vi "goInCircles.vi"(8 "error in (no error)":errorcluster, 11 "StationKeeping in":refnum<class "StationKeeping.lvclass">) -> (0 "error out":errorcluster, 2 "No Sail Circles":T1[](array[typedef]), 3 "StationKeeping out":refnum<class "StationKeeping.lvclass">)   [LabVIEW 2011, in "StationKeeping.lvclass"]
uses:
  StationKeeping.lvclass
  2 Typedefs/UTM Circle.ctl
  StationKeeping.lvclass/StationKeeping.ctl
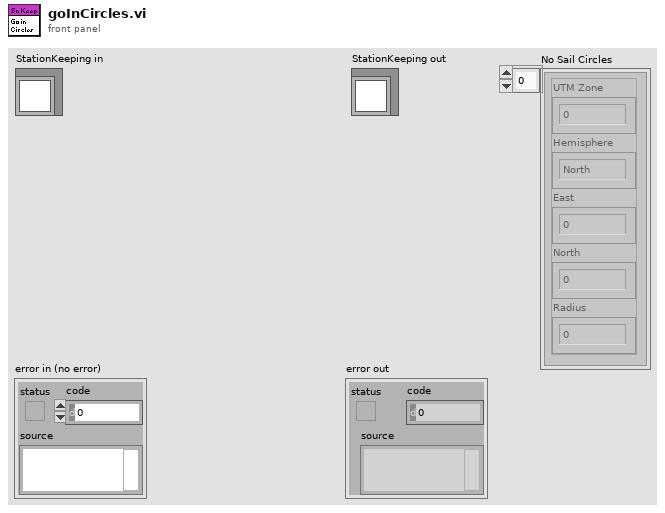
[diagram p1: front panel]
types:
  T1 = typedef "UTM Circle.ctl" = cluster{"UTM Zone":dbl, "Hemisphere":enum16{"North", "South"}, "East":dbl, "North":dbl, "Radius":dbl}
  T2 = typedef "UTM Location.ctl" = cluster{"UTM Zone":dbl, "Hemisphere":enum16{"North", "South"}, "East":dbl, "North":dbl}
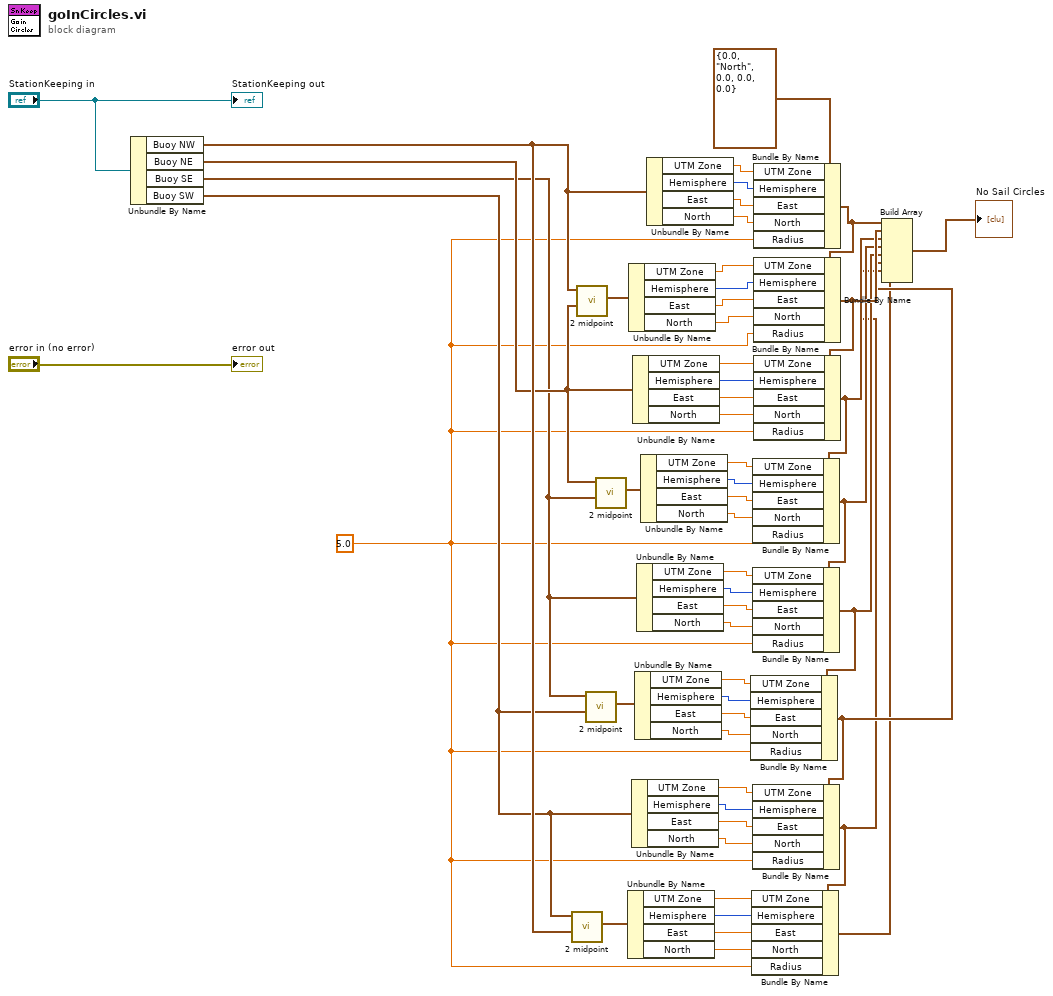
[diagram p0: block diagram]
diagram:
  w1 = 5.0 ("Radius")
  n1 = Unbundle By Name("StationKeeping in") -> ("Buoy NW"=w5:T2, "Buoy NE"=w4:T2, "Buoy SE"=w3:T2, "Buoy SW"=w2:T2)
  n2 = call "2 midpoint.vi"("UTM 2"=w5, "UTM 1"=w2) -> ("Midpoint"=w10:T2)  [unwired: 8 in, 1 out]
  n3 = call "2 midpoint.vi"("UTM 2"=w4, "UTM 1"=w5) -> ("Midpoint"=w7:T2)  [unwired: 8 in, 1 out]
  n4 = call "2 midpoint.vi"("UTM 2"=w2, "UTM 1"=w3) -> ("Midpoint"=w9:T2)  [unwired: 8 in, 1 out]
  n5 = call "2 midpoint.vi"("UTM 2"=w3, "UTM 1"=w4) -> ("Midpoint"=w8:T2)  [unwired: 8 in, 1 out]
  n6 = Unbundle By Name(w10) -> ("UTM Zone"=w31:dbl, "Hemisphere"=w32:enum16{"North", "South"}, "East"=w33:dbl, "North"=w34:dbl)
  n7 = Unbundle By Name(w7) -> ("UTM Zone"=w38:dbl, "Hemisphere"=w37:enum16{"North", "South"}, "East"=w36:dbl, "North"=w35:dbl)
  n8 = Unbundle By Name(w2) -> ("UTM Zone"=w27:dbl, "Hemisphere"=w28:enum16{"North", "South"}, "East"=w29:dbl, "North"=w30:dbl)
  n9 = Unbundle By Name(w4) -> ("UTM Zone"=w11:dbl, "Hemisphere"=w12:enum16{"North", "South"}, "East"=w13:dbl, "North"=w14:dbl)
  n10 = Unbundle By Name(w9) -> ("UTM Zone"=w23:dbl, "Hemisphere"=w24:enum16{"North", "South"}, "East"=w25:dbl, "North"=w26:dbl)
  n11 = Unbundle By Name(w3) -> ("UTM Zone"=w19:dbl, "Hemisphere"=w20:enum16{"North", "South"}, "East"=w21:dbl, "North"=w22:dbl)
  n12 = Unbundle By Name(w8) -> ("UTM Zone"=w15:dbl, "Hemisphere"=w16:enum16{"North", "South"}, "East"=w17:dbl, "North"=w18:dbl)
  n13 = Unbundle By Name(w5) -> ("UTM Zone"=w50:dbl, "Hemisphere"=w49:enum16{"North", "South"}, "East"=w48:dbl, "North"=w47:dbl)
  n14 = Bundle By Name(cluster=T1 {"UTM Zone"=0.0, "Hemisphere"=enum."North", "East"=0.0, "North"=0.0, "Radius"=0.0} ("UTM Location"), "UTM Zone"=w50, "Hemisphere"=w49, "East"=w48, "North"=w47, "Radius"=w1) -> (w46:T1)
  n15 = Bundle By Name(cluster=w46, "UTM Zone"=w38, "Hemisphere"=w37, "East"=w36, "North"=w35, "Radius"=w1) -> (w45:T1)
  n16 = Bundle By Name(cluster=w45, "UTM Zone"=w11, "Hemisphere"=w12, "East"=w13, "North"=w14, "Radius"=w1) -> (w44:T1)
  n17 = Bundle By Name(cluster=w44, "UTM Zone"=w15, "Hemisphere"=w16, "East"=w17, "North"=w18, "Radius"=w1) -> (w43:T1)
  n18 = Bundle By Name(cluster=w43, "UTM Zone"=w19, "Hemisphere"=w20, "East"=w21, "North"=w22, "Radius"=w1) -> (w42:T1)
  n19 = Bundle By Name(cluster=w42, "UTM Zone"=w23, "Hemisphere"=w24, "East"=w25, "North"=w26, "Radius"=w1) -> (w41:T1)
  n20 = Bundle By Name(cluster=w41, "UTM Zone"=w27, "Hemisphere"=w28, "East"=w29, "North"=w30, "Radius"=w1) -> (w39:T1)
  n21 = Bundle By Name(cluster=w39, "UTM Zone"=w31, "Hemisphere"=w32, "East"=w33, "North"=w34, "Radius"=w1) -> (w40:T1)
  n22 = Build Array(w46, w45, w44, w43, w42, w41, w39, w40) -> (→"No Sail Circles":T1[])
  "error out" <- "error in (no error)"
  "StationKeeping out" <- "StationKeeping in"
